vi "liblinear_predict_probability.vi"(8 "error in (no error)":errorcluster, 10 "x":T1[](array[typedef]), 11 "liblinear_model":T2={"liblinear_parameter"={"solver_type"=0, "eps"=0.01, "C"=1.0, "weight_label"=[], "weight"=[], "p"=0.1}, "nr_class"=0, "nr_feature"=0, "w"=[], "label"=[], "bias"=0.0} {"liblinear_parameter"."solver_type" items=["L2R_LR"=0, "L2R_L2LOSS_SVC_DUAL"=1, "L2R_L2LOSS_SVC"=2, "L2R_L1LOSS_SVC_DUAL"=3, "MCSVM_CS"=4, "L1R_L2LOSS_SVC"=5, "L1R_LR"=6, "L2R_LR_DUAL"=7, "L2R_L2LOSS_SVR"=11, "L2R_L2LOSS_SVR_DUAL"=12, "L2R_L1LOSS_SVR_DUAL"=13]}) -> (0 "error out":errorcluster, 2 "Probability estimates":dbl[](array[numeric]), 3 "Predicted label":dbl)   [LabVIEW 2015]
uses:
  Controls/liblinear_model.ctl
  Controls/liblinear_parameter.ctl
  Controls/liblinear_solver.ctl
  LibSVM Sparse/Wrapper API/Controls/svm_node.ctl
  bin/x64/LabVIEW-liblinear.dll
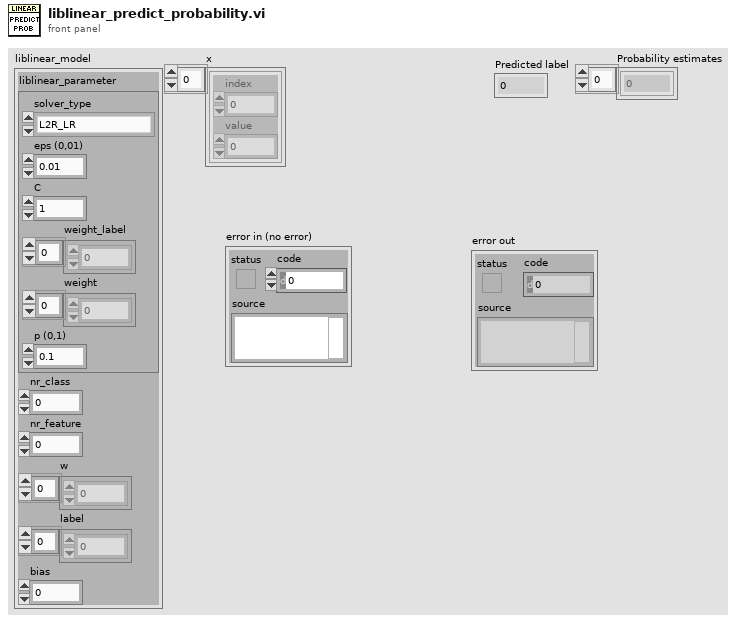
[diagram p1: front panel]
types:
  T1 = typedef "svm_node.ctl" = cluster{"index":i32, "value":dbl}
  T2 = typedef "liblinear_model.ctl" = cluster{"liblinear_parameter":T3, "nr_class":i32, "nr_feature":i32, "w":dbl[], "label":i32[], "bias":dbl}
  T3 = typedef "liblinear_parameter.ctl" = cluster{"solver_type":T4, "eps":dbl, "C":dbl, "weight_label":i32[], "weight":dbl[], "p":dbl}
  T4 = typedef "liblinear_solver.ctl" = u32
  T5 = typedef "svm_node_padded.ctl" = cluster{"index":i32, "padding":i32, "value":dbl}
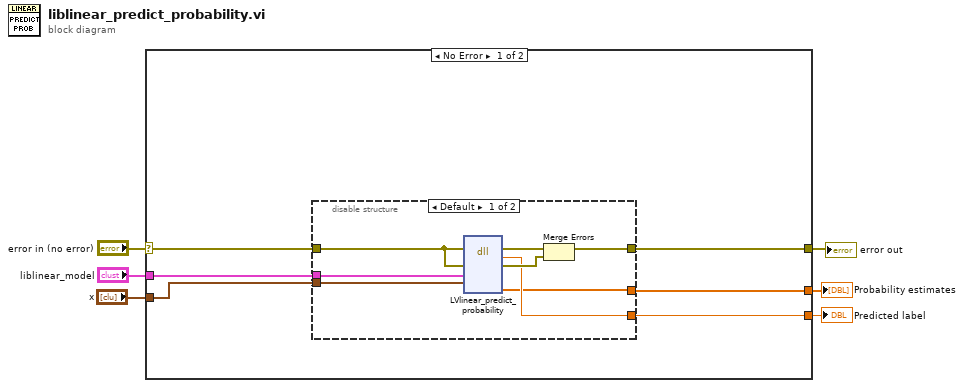
[diagram p0: block diagram]
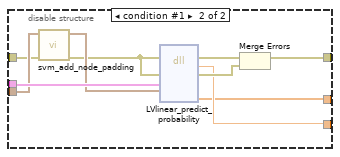
[diagram p2: hidden frame]
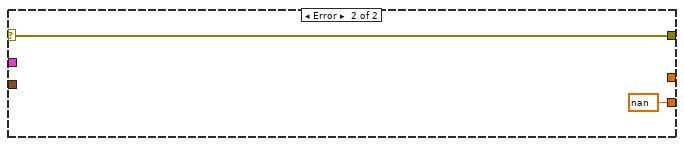
[diagram p3: hidden frame]
diagram:
  n1 = case shown="No Error" "error in (no error)" {
    selector: "error in (no error)" -> [w12 w32]
    tunnel: [w11 w32] -> w6
    tunnel: "liblinear_model" -> [w10 _]
    tunnel: "x" -> [w9 _]
    tunnel: [w8 nan ("predicted label")] -> w2
    tunnel: [w7 _] -> w1
    frame No Error {
      n2 = disable-structure shown="Default" {
        disable-tunnel: w12 -> [w20 w22]
        disable-tunnel: [w18 w29] -> w11
        disable-tunnel: w10 -> [w16 w27]
        disable-tunnel: w9 -> [w15 w24]
        disable-tunnel: [w14 w26] -> w8
        disable-tunnel: [w13 w25] -> w7
        frame condition #0 (active) {
          n3 = dll-call lib="C:/dev/LabVIEW-libsvm/LabVIEW/bin/x64/LabVIEW-liblinear.*" fn="LVlinear_predict_probability"(error in=w20, "lvErr"=w20, "model_in"=w16, "x_in"=w15) -> (error out=w19:errorcluster, "predicted label"=w14:dbl, "lvErr"=w17:errorcluster, "prob_estimates_out"=w13:dbl[])  [unwired: 5 in, 1 out]
          n4 = Merge Errors(w19, w17) -> (w18:errorcluster)
        }
        frame condition #1 {
          n5 = call "svm_add_node_padding.vi"("error in (no error)"=w22, "Nodes"=w24) -> ("error out"=w21:errorcluster, "Padded nodes"=w23:T5[])  [unwired: 8 in]
          n6 = dll-call lib="C:/dev/LabVIEW-libsvm/LabVIEW/bin/x64/LabVIEW-liblinear.*" fn="LVlinear_predict_probability"(error in=w21, "lvErr"=w21, "model_in"=w27, "x_in"=w23) -> (error out=w30:errorcluster, "predicted label"=w26:dbl, "lvErr"=w28:errorcluster, "prob_estimates_out"=w25:dbl[])  [unwired: 5 in, 1 out]
          n7 = Merge Errors(w30, w28) -> (w29:errorcluster)
        }
      }
    }
    frame Error {
    }
  }
  "error out" <- w6
  "Predicted label" <- w2
  "Probability estimates" <- w1
